vi "Log MCLI Configuration.vi"(8 "error in (no error)":errorcluster, 11 "Instrument.Lockin in":refnum<class "Instrument.Lockin.lvclass">) -> (0 "error out":errorcluster, 3 "Instrument.Lockin out":refnum<class "Instrument.Lockin.lvclass">)   [LabVIEW 2019, in "Instrument.Lockin.lvlib" / "Instrument.Lockin.lvclass"]
uses:
  Instrument.Lockin.lvclass
  <userlib>/LevyLab/Instrument Framework/Instrument/Instrument.lvclass
  C:/Program Files/National Instruments/LabVIEW 2019/user.lib/LevyLab/Instrument Framework/Instrument Types/Lockin/Instrument.LockinAPI.lvclass
  C:/Program Files/National Instruments/LabVIEW 2019/user.lib/LevyLab/Instrument Framework/Instrument/Instrument.lvclass
  C:/Program Files/National Instruments/LabVIEW 2019/vi.lib/JKI/JKI SMO/SMO/SMO.lvclass
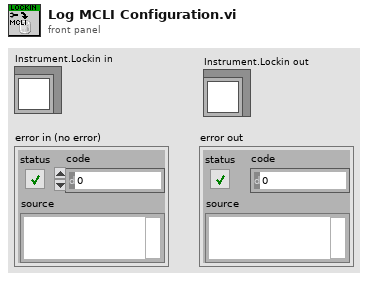
[diagram p1: front panel]
types:
  T1 = typedef "Instrument.Lockin.lvlib/Instrument.Lockin.lvclass/Lockin.LogConfiguration.MCLI--Cluster.ctl" = cluster{"System Serial Number":string, "Software Version":string, "REF Channel":i32, "frequency":dbl, "time constant":dbl, "roll-off":i32}
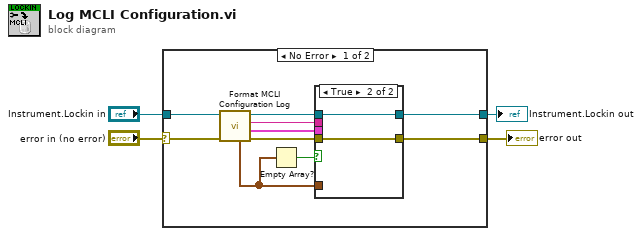
[diagram p0: block diagram]
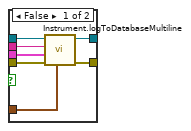
[diagram p2: hidden frame]
diagram:
  n1 = case shown="No Error" "error in (no error)" {
    selector: "error in (no error)" -> [w14 w25]
    tunnel: "Instrument.Lockin in" -> [w13 w24]
    tunnel: [w6 w25] -> w3
    tunnel: [w5 w24] -> w1
    frame No Error {
      n2 = call "Format MCLI Configuration Log.vi"("error in (no error)"=w14, "Instrument.Lockin in"=w13) -> ("error out"=w9:errorcluster, "Log Data"=w10:T1[], "Log Paths"=w11:string, "Instrument.Lockin out"=w12:refnum<class "Instrument.Lockin.lvclass">, "Times"=w7:timestamp[])  [unwired: 5 in]
      n3 = Empty Array?(array=w7) -> (empty?=w8:bool)
      n4 = case shown="True" w8 {
        tunnel: [w21 w23] -> w6
        tunnel: [w20 w22] -> w5
        tunnel: w12 -> [w19 w22]
        tunnel: w11 -> [w18 _]
        tunnel: w10 -> [w17 _]
        tunnel: w7 -> [w16 _]
        tunnel: w9 -> [w15 w23]
        frame False {
          n5 = call <userlib>:"Instrument.logToDatabaseMultiline.vi"("timestamps"=w16, "error in (no error)"=w15, "Data"=w17, "Paths"=w18, "Instrument"=w19) -> ("error out"=w21:errorcluster, "Instrument out"=w20:refnum<class "Instrument.Lockin.lvclass">)  [unwired: 5 in]
        }
        frame True {
        }
      }
    }
    frame Error {
    }
  }
  "error out" <- w3
  "Instrument.Lockin out" <- w1
